vi "Set dcvmDPI Configure.vi"(7 "Streaming? (F)":bool, 8 "error in (no error)":errorcluster, 10 "Message Data":T1, 11 "gRPCid in":T3) -> (0 "error out":errorcluster)   [LabVIEW 2021, in "dcvmDPI_AD7606B_server.lvlib" / "dcvmDPI.lvclass"]
uses:
  dcvmDPI.lvclass
  <vilib>/gRPC/LabVIEW gRPC Library/Shared/grpcId.ctl
  RPC Messages/dcvmDPI_ConfigureResponse.ctl
  RPC Messages/dcvmDPI_ErrorResponse.ctl
  dcvmDPI.lvclass/dcvmDPI.ctl
  dcvmDPI_AD7606B_server.lvlib
  <vilib>/gRPC/LabVIEW gRPC Library/grpc-lvsupport-release.lvlib
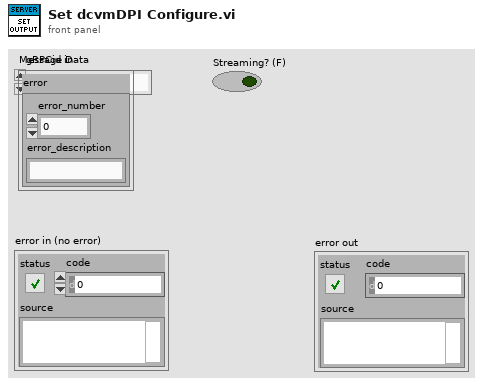
[diagram p1: front panel]
types:
  T1 = typedef "dcvmDPI_AD7606B_server.lvlib/dcvmDPI_ConfigureResponse.ctl" = cluster{"error":T2}
  T2 = typedef "dcvmDPI_AD7606B_server.lvlib/dcvmDPI_ErrorResponse.ctl" = cluster{"error_number":i32, "error_description":string}
  T3 = typedef "grpc-lvsupport-release.lvlib/grpcId.ctl" = u64
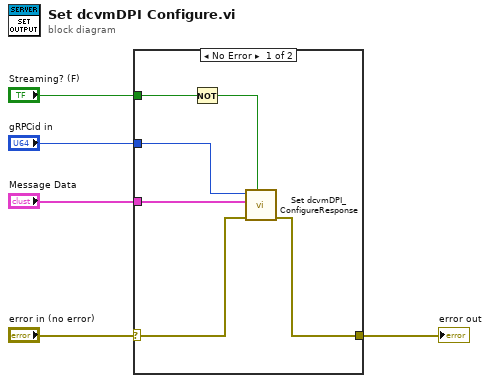
[diagram p0: block diagram]
diagram:
  n1 = case shown="No Error" "error in (no error)" {
    selector: "error in (no error)" -> [w11 w12]
    tunnel: [w9 w12] -> w4
    tunnel: "gRPCid in" -> [w10 _]
    tunnel: "Message Data" -> [w8 _]
    tunnel: "Streaming? (F)" -> [w7 _]
    frame No Error {
      n2 = Not(x=w7) -> (.not. x?=w6:bool)
      n3 = call "Set dcvmDPI_ConfigureResponse.vi"("Complete Call (T)"=w6, "error in (no error)"=w11, "package_templatemessage"=w8, "gRPCid"=w10) -> ("error out"=w9:errorcluster)  [unwired: 7 in]
    }
    frame Error {
    }
  }
  "error out" <- w4
